vi "Initialize_automation_setup.vi"() -> ()   [LabVIEW 2017]
panel:
  out "Test verdict":string
  out "Test Result":picture
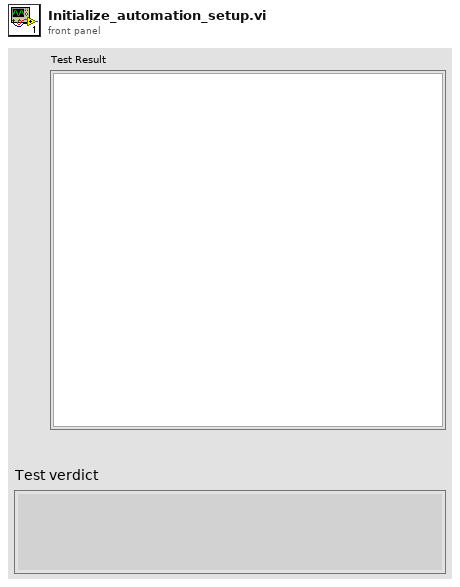
[diagram p1: front panel]
types:
  T1 = enum16{"open", "replace", "create", "open or create", "replace or create", "replace or create with confirmation"}
  T2 = cluster{"[0]":string, "[1]":string, "[2]":string, "[3]":string, "[4]":string, "[5]":string, "[6]":string, "[7]":string, "[8]":string}
  T3 = cluster{"Socket_IP_Address":string, "Socket_Port_Number":u16, "Global_ReportPath":path}
  T4 = cluster{"Iterations":u64, "DelayBetweenIterations":u32, "Timeout":u32, "MessageID":i32, "MessageLength":i32, "ResponseID":i32, "Timestamp":string, "TestSuite":string, "ReportPath":path, "FWVersionPath":path}
  T5 = typedef "imagedata.ctl" = cluster{"image type":i32, "image depth":i32, "image":u8[], "mask":u8[], "colors":u32[], "Rectangle":cluster{"left":i16, "top":i16, "right":i16, "bottom":i16}}
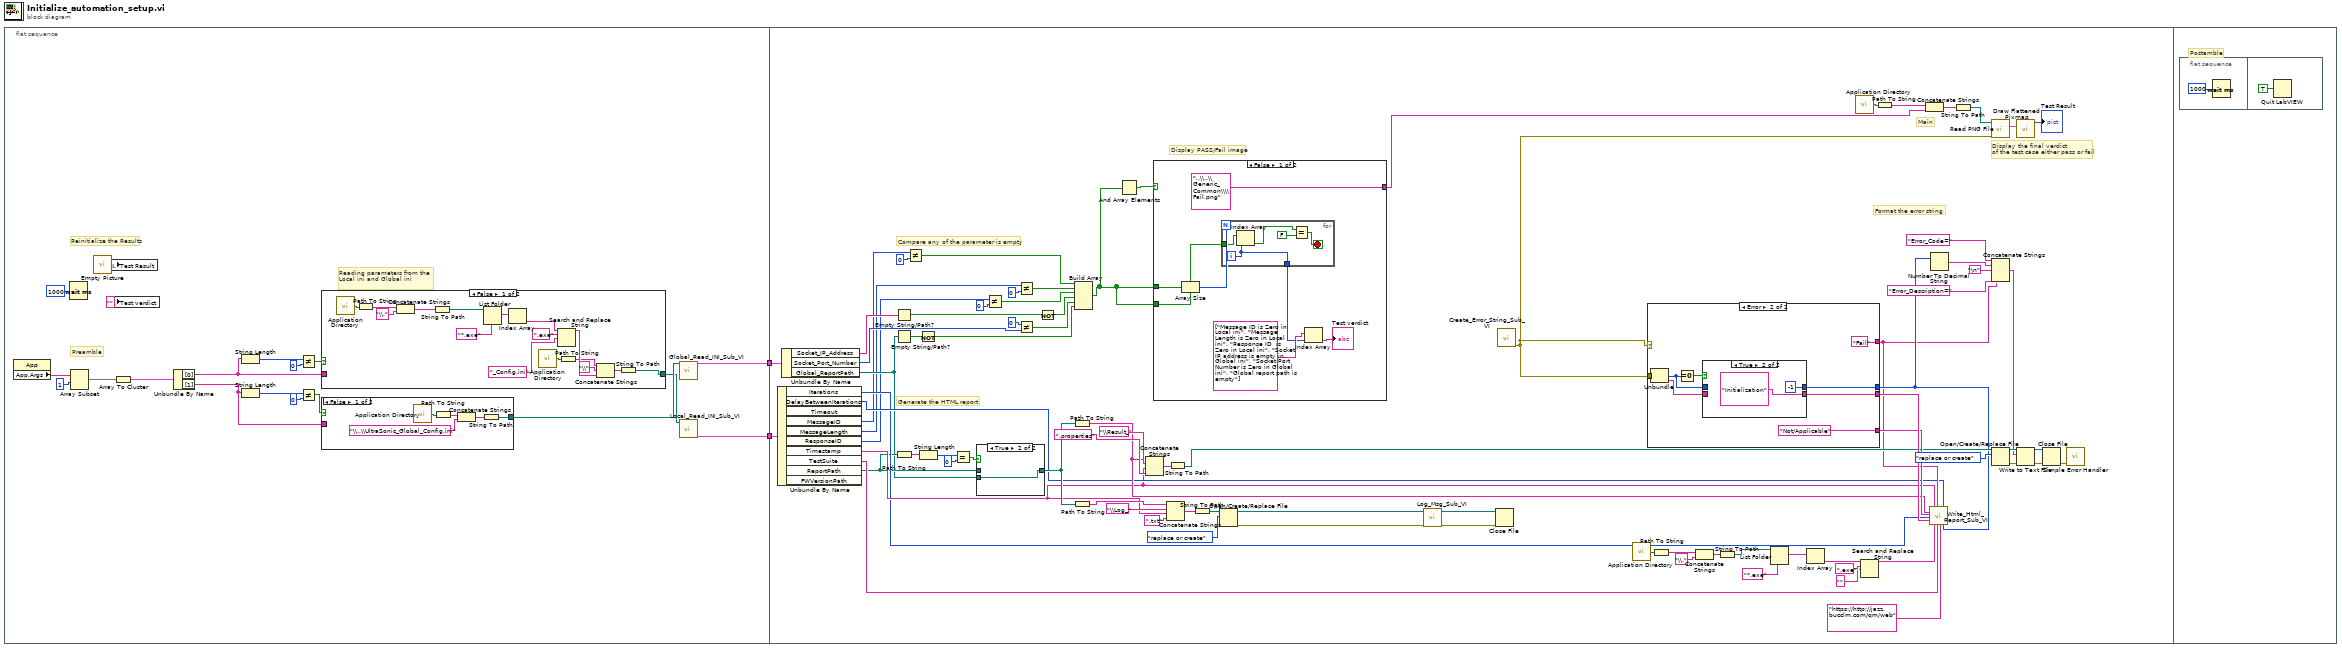
[diagram p0: block diagram]
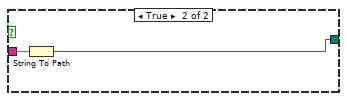
[diagram p2: hidden frame]
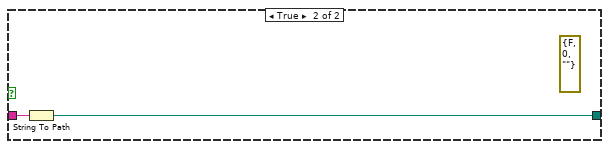
[diagram p3: hidden frame]
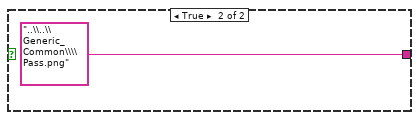
[diagram p4: hidden frame]
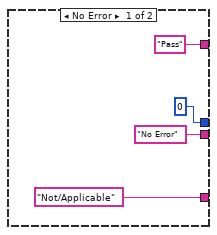
[diagram p6: hidden frame]
diagram:
  n1 = flat-sequence {
    tunnel: [w7] -> w2
    tunnel: [w6] -> w1
    tunnel: w2 -> [w75]
    tunnel: w1 -> [w69]
    frame #0 {
      # "Reinitialize the Results"
      # "Reading parameters from the\nLocal ini and Global ini"
      # "Preamble"
      n2 = property class="App"() -> ("App.Args"=w9:string[])  [unwired: 2 in, 2 out]
      n3 = Wait (ms)(milliseconds to wait=u32 1000) -> ()  [unwired: 1 out]
      n4 = Array Subset "Array Subset"(array=w9, index=1) -> (w10:string[])  [unwired: 1 in]
      n5 = call "Empty Picture"() -> ("empty picture"=w4:picture)
      n6 = local write "Test Result"(w4) -> ()
      n7 = local write "Test verdict"("" ("String")) -> ()
      n8 = Array To Cluster(array=w10) -> (cluster=w11:T2)
      n9 = Unbundle By Name "Unbundle By Name"(w11) -> ("[0]"=w15:string, "[1]"=w18:string)
      n10 = String Length(string=w15) -> (length=w12:i32)
      n11 = String Length(string=w18) -> (length=w19:i32)
      n12 = Not Equal?(x=w12, y=0) -> (x != y?=w14:bool)
      n13 = Not Equal?(x=w19, y=0) -> (x != y?=w17:bool)
      n14 = case shown="False" w14 {
        tunnel: w15 -> [_ w46]
        tunnel: [w29 w45] -> w20
        frame False {
          n15 = call <vilib>:"Application Directory.vi"() -> ("Application Directory"=w35:path)
          n16 = Path To String(path=w35) -> (string=w34:string)
          n17 = Concatenate Strings(w34, "\\." ("string")) -> (w32:string)
          n18 = String To Path(string=w32) -> (path=w37:path)
          n19 = List Folder(path=w37, pattern="*.exe") -> (filenames=w31:string[])  [unwired: 2 in, 3 out]
          n20 = Index Array(array=w31) -> (element=w30:string)  [unwired: 1 in]
          n21 = call <vilib>:"Application Directory.vi"() -> ("Application Directory"=w44:path)
          n22 = Search and Replace String(input string=w30, search string=".exe", replace string="_Config.ini" ("replace string (\"\")")) -> (result string=w41:string)  [unwired: 5 in, 3 out]
          n23 = Path To String(path=w44) -> (string=w39:string)
          n24 = Concatenate Strings(w39, "\\" ("string"), w41) -> (w38:string)
          n25 = String To Path(string=w38) -> (path=w29:path)
        }
        frame True {
          (unwired) errorcluster {"status"=FALSE, "code"=0, "source"=""} ("error out")
          n26 = String To Path(string=w46) -> (path=w45:path)
        }
      }
      n27 = case shown="False" w17 {
        tunnel: [w23 w28] -> w21
        tunnel: w18 -> [_ w27]
        frame False {
          n28 = call <vilib>:"Application Directory.vi"() -> ("Application Directory"=w22:path)
          n29 = Path To String(path=w22) -> (string=w26:string)
          n30 = Concatenate Strings(w26, "\\..\\UltraSonic_Global_Config.ini" ("string")) -> (w24:string)
          n31 = String To Path(string=w24) -> (path=w23:path)
        }
        frame True {
          n32 = String To Path(string=w27) -> (path=w28:path)
        }
      }
      n33 = call "Global_Read_INI_Sub_VI.vi"("Config File Path"=w21) -> ("output cluster"=w7:T3)  [unwired: 14 in]
      n34 = call "Local_Read_INI_Sub_VI.vi"("Config File Path"=w20) -> ("output cluster"=w6:T4)  [unwired: 10 in]
    }
    frame #1 {
      # "Display PASS/Fail image"
      # "Generate the HTML report"
      # "Display the final verdict \nof the test case either pass or fail"
      # "Format the error string"
      # "Compare any of the parameter is empty"
      # "Main"
      n35 = Unbundle By Name(w69) -> ("Iterations"=w71:u64, "DelayBetweenIterations"=w74:u32, "MessageID"=w64:i32, "MessageLength"=w63:i32, "ResponseID"=w62:i32, "Timestamp"=w73:string, "TestSuite"=w72:string, "ReportPath"=w70:path)  [unwired: 2 out]
      n36 = Unbundle By Name(w75) -> ("Socket_IP_Address"=w66:string, "Socket_Port_Number"=w68:u16, "Global_ReportPath"=w65:path)
      n37 = Empty String/Path?(string/path=w66) -> (empty?=w54:bool)
      n38 = Empty String/Path?(string/path=w65) -> (empty?=w52:bool)
      n39 = Path To String(path=w70) -> (string=w120:string)
      n40 = Not Equal?(x=w64, y=0) -> (x != y?=w58:bool)
      n41 = Not(x=w52) -> (.not. x?=w51:bool)
      n42 = String Length(string=w120) -> (length=w119:i32)
      n43 = Equal?(x=w119, y=0) -> (x = y?=w117:bool)
      n44 = case shown="True" w117 {
        tunnel: w65 -> [_ w143]
        tunnel: [w142 w143] -> w116
        tunnel: w70 -> [w142 _]
        frame False {
        }
        frame True {
        }
      }
      n45 = Not Equal?(x=w62, y=0) -> (x != y?=w56:bool)
      n46 = Not Equal?(x=w63, y=0) -> (x != y?=w57:bool)
      n47 = Not Equal?(x=u16 0, y=w68) -> (x != y?=w55:bool)
      n48 = Not(x=w54) -> (.not. x?=w53:bool)
      n49 = Path To String(path=w116) -> (string=w93:string)
      n50 = Path To String(path=w116) -> (string=w122:string)
      n51 = Build Array(w58, w57, w56, w53, w55, w51) -> (w47:bool[])
      n52 = And Array Elements(Boolean array=w47) -> (logical AND=w49:bool)
      n53 = Concatenate Strings(w93, "\\Result_" ("string"), w73, ".properties" ("string")) -> (w114:string)
      n54 = case shown="False" w49 {
        tunnel: ["..\\..\\Generic_Common\\\\Fail.png" ("string") "..\\..\\Generic_Common\\\\Pass.png" ("string")] -> w48
        tunnel: w47 -> [w134 _]
        tunnel: w47 -> [w132 _]
        frame False {
          n55 = Array Size(array=w134) -> (size(s)=w133:i32)
          n56 = for {
            N: w133 -> [_]
            tunnel: w132 -> [w140]
            tunnel: [w137] -> w130
            i -> [w137]
            stop <- w136 stop-if-true
            n57 = Index Array(array=w140, index=w137) -> (element=w139:bool)
            n58 = Equal?(x=w139, y=FALSE) -> (x = y?=w136:bool)
          }
          n59 = Index Array(array=string[] ["Message ID is Zero in Local ini", "Message Length is Zero in Local ini", "Response ID  is Zero in Local ini", "Socket IP address is empty in Global ini", "Socket Port Number is Zero in Global ini", "Global report path is empty"], index=w130) -> (element=→"Test verdict":string)
        }
        frame True {
        }
      }
      n60 = Concatenate Strings(w122, "\\Log_" ("string"), w73, ".txt" ("string")) -> (w125:string)
      n61 = String To Path(string=w114) -> (path=w106:path)
      n62 = String To Path(string=w125) -> (path=w124:path)
      n63 = Open/Create/Replace File(file path (use dialog)=w124, operation (0:open)=T1."replace or create") -> (refnum out=w94:refnum<file>, error out=w97:errorcluster)  [unwired: 1 in, 4 out]
      n64 = call "Log_Msg_Sub_VI.vi"("error in (no error)"=w97, "Byte Stream File in"=w94) -> ("error out"=w95:errorcluster, "Byte Stream File out"=w96:refnum<file>)  [unwired: 8 in]
      n65 = Close File(refnum=w96, error in=w95) -> ()  [unwired: 2 out]
      n66 = call "Create_Error_String_Sub_VI.vi"() -> ("error out"=w50:errorcluster)  [unwired: 10 in, 1 out]
      n67 = call <vilib>:"Application Directory.vi"() -> ("Application Directory"=w90:path)
      n68 = case shown="Error" w50 {
        tunnel: ["Pass" "Fail"] -> w98
        tunnel: w50 -> [_ w153]
        tunnel: [0 ("code") w150] -> w102
        tunnel: ["No Error" ("source") w151] -> w128
        tunnel: ["Not/Applicable" "Not/Applicable"] -> w127
        frame No Error {
        }
        frame Error {
          n69 = Unbundle(w153) -> ("code"=w152:i32, "source"=w148:string)  [unwired: 1 out]
          n70 = Equal To 0?(x=w152) -> (x = 0?=w149:bool)
          n71 = case shown="True" w149 {
            tunnel: [w157 -1 ("code")] -> w150
            tunnel: [w156 "Initialization" ("source")] -> w151
            tunnel: w152 -> [w157 _]
            tunnel: w148 -> [w156 _]
            frame False {
            }
            frame True {
            }
          }
        }
      }
      n72 = Path To String(path=w90) -> (string=w89:string)
      n73 = Concatenate Strings(w89, "\\." ("string")) -> (w87:string)
      n74 = String To Path(string=w87) -> (path=w92:path)
      n75 = List Folder(path=w92, pattern="*.exe") -> (filenames=w86:string[])  [unwired: 2 in, 3 out]
      n76 = Index Array(array=w86) -> (element=w82:string)  [unwired: 1 in]
      n77 = call <vilib>:"Application Directory.vi"() -> ("Application Directory"=w76:path)
      n78 = Search and Replace String(input string=w82, search string=".exe", replace string="" ("replace string (\"\")")) -> (result string=w85:string)  [unwired: 5 in, 3 out]
      n79 = Path To String(path=w76) -> (string=w77:string)
      n80 = Concatenate Strings(w77, w48) -> (w78:string)
      n81 = call "Write_Html_Report_Sub_VI.vi"("ReprtPath"=w93, "Remarks"=w127, "Iterations"=w71, "Error Description"=w128, "Timestamp"=w73, "TestCase"=w85, "Verdict"=w98, "TestSuite"=w72, "JazzDashboardLink"="https://http://jazz.bucclm.com/qm/web" ("TestSuite"), "Delay Between Iterations"=w74, "Error Code"=w102) -> ()  [unwired: 9 in]
      n82 = Number To Decimal String(number=w102) -> (decimal integer string=w101:string)  [unwired: 1 in]
      n83 = String To Path(string=w78) -> (path=w81:path)
      n84 = call <vilib>:"Read PNG File.vi"("error in (no error)"=w50, "path to PNG file"=w81) -> ("image data"=w79:T5)  [unwired: 7 in, 2 out]
      n85 = Concatenate Strings("Error_Code=" ("string"), w101, "\n", "Error_Description=" ("string"), w98) -> (w104:string)
      n86 = Open/Create/Replace File(file path (use dialog)=w106, operation (0:open)=T1."replace or create") -> (refnum out=w105:refnum<file>, error out=w110:errorcluster)  [unwired: 4 in, 1 out]
      n87 = call <vilib>:"Draw Flattened Pixmap.vi"("image data"=w79) -> ("new picture"=→"Test Result":picture)  [unwired: 8 in]
      n88 = Write to Text File(file (use dialog)=w105, text=w104, error in=w110) -> (refnum out=w109:refnum<file>, error out=w108:errorcluster)  [unwired: 1 in, 1 out]
      n89 = Close File(refnum=w109, error in=w108) -> (error out=w107:errorcluster)  [unwired: 1 out]
      n90 = call <vilib>:"Simple Error Handler.vi"("error in (no error)"=w107) -> ()  [unwired: 4 in, 5 out]
    }
    frame #2 {
      # "Postamble"
      n91 = flat-sequence {
        frame #0 {
          n92 = Wait (ms)(milliseconds to wait=u32 1000) -> ()  [unwired: 1 out]
        }
        frame #1 {
          n93 = Quit LabVIEW(quit? (T)=TRUE) -> ()
        }
      }
    }
  }
